vi "Create Table.vi"(0 "database in":path, 1 "Table name in":string, 5 "Column Names":string[](array[string]), 7 "Columns Type Affinity":enum16{"TEXT", "NUM", "INT", "REAL", "BLOB"}[](array[ring]), 9 "Additional constraints":string[](array[string]), 11 "error in (no error)":errorcluster) -> (15 "error out":errorcluster)   [LabVIEW 2020, in "sqlite3.lvlib"]
uses:
  sqlite3.lvlib
  sqlite/VIs/open v2.vi
  sqlite/VIs/prepare v2.vi
  sqlite/VIs/step.vi
  sqlite/VIs/column count.vi
  compound/Column.vi
  compound/Resolve Result Type.vi
  sqlite/VIs/finalize.vi
  sqlite/VIs/close v2.vi
  sqlite/subvi/Error Converter (ErrCode or Status).vi
  sqlite/VIs/column text.vi
  sqlite/VIs/column bytes.vi
  sqlite/VIs/column blob.vi
  utilities/MoveBlock.vi
  sqlite/VIs/column type.vi
  sqlite/VIs/errstr.vi
panel:
  out "SQL out":string="CREATE TABLE IF NOT EXISTS test (a INT PRIMARY KEY, name TEXT , temperature REAL , image BLOB , encounters NUM );"
  # "mixed feelings about\nquery helper vis\n\non one hand, they can make \nsimple queries even easier\n\notoh, they can limit options and dev knowledge\ndue to the breadth of SQL options\navailable, nothing short of re-implementing\nall the sql query parsing rules would be enough"
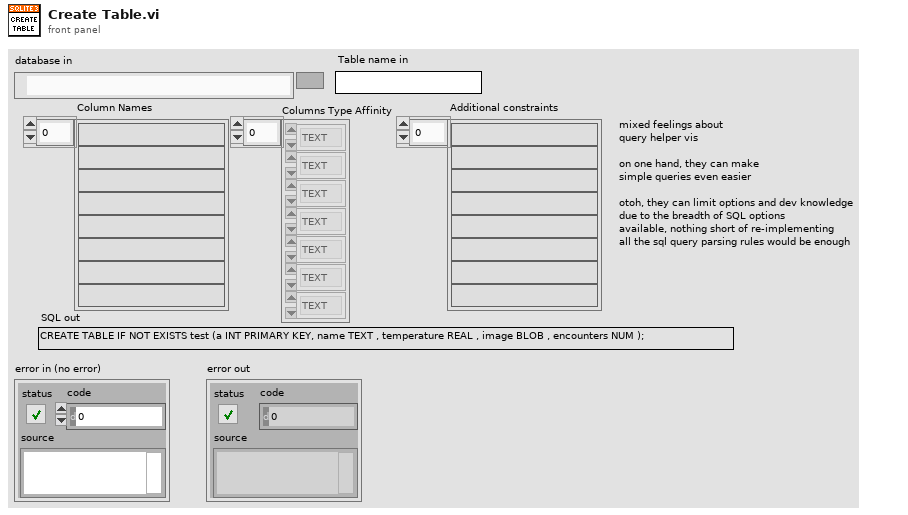
[diagram p1: front panel]
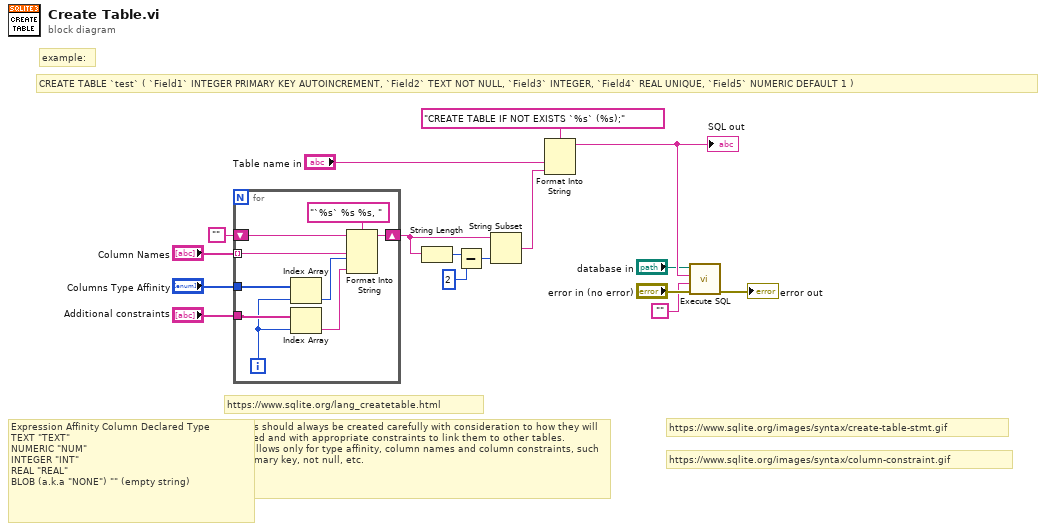
[diagram p0: block diagram]
diagram:
  # "example:"
  # "CREATE TABLE `test` ( `Field1` INTEGER PRIMARY KEY AUTOINCREMENT, `Field2` TEXT NOT NULL, `Field3` INTEGER, `Field4` REAL UNIQUE, `Field5` NUMERIC DEFAULT 1 )"
  # "https://www.sqlite.org/images/syntax/create-table-stmt.gif"
  # "https://www.sqlite.org/images/syntax/column-constraint.gif"
  # "Tables should always be created carefully with consideration to how they will be used and with appropriate constraints to link them to other tables.\nThis allows only for type affinity, column names and column constraints, such as primary key, not null, etc."
  # "https://www.sqlite.org/lang_createtable.html"
  # "Expression Affinity\tColumn Declared Type\nTEXT\t\"TEXT\"\nNUMERIC\t\"NUM\"\nINTEGER\t\"INT\"\nREAL\t\"REAL\"\nBLOB (a.k.a \"NONE\")\t\"\" (empty string)"
  n1 = for {
    tunnel: "Column Names" -> [w25] mode=indexing
    tunnel: "Columns Type Affinity" -> [w21]
    tunnel: "Additional constraints" -> [w19]
    shift-right: [w23] -> w9
    shift-left: "" -> [w22]
    i -> [w18]
    n2 = Index Array(array=w21, index=w18) -> (element=w20:enum16{"TEXT", "NUM", "INT", "REAL", "BLOB"})
    n3 = Index Array(array=w19, index=w18) -> (element=w17:string)
    n4 = Format Into String(format string="`%s` %s %s, ", initial string=w22, w25, w20, w17) -> (resulting string=w23:string)  [unwired: 1 in, 1 out]
  }
  n5 = String Length(string=w9) -> (length=w7:i32)
  n6 = Subtract(x=w7, y=2 ("x")) -> (x-y=w6:i32)
  n7 = String Subset(string=w9, length (rest)=w6) -> (substring=w8:string)  [unwired: 1 in]
  n8 = Format Into String(format string="CREATE TABLE IF NOT EXISTS `%s` (%s);", "Table name in", w8) -> (resulting string=w10:string)  [unwired: 2 in, 1 out]
  "SQL out" <- w10
  n9 = call "Execute SQL.vi"("error in (no error)"="error in (no error)", "[disabled] return type (string)"="", "sql (string)"=w10, "database in"="database in") -> ("error out"=→"error out":errorcluster)  [unwired: 6 in, 1 out]
